vi "ForecastData Randomize Short.vi"(10 "DeviceID":T2) -> (3 "ForecastData_Short Array out":T1[](array[typedef]))   [LabVIEW 2018, in "IED Test Framework.lvlib" / "IED Test.lvclass"]
uses:
  IED Test.lvclass
  <vilib>/ORNL/CSEISMIC DDS/CSEISMIC DDS Base/Data Types/Controls/DeviceID.ctl
  <vilib>/ORNL/CSEISMIC DDS/CSEISMIC DDS Base/Data Types/ForecastData_Data.ctl
  <vilib>/ORNL/CSEISMIC DDS/CSEISMIC DDS Base/CSEISMIC DDS.lvclass
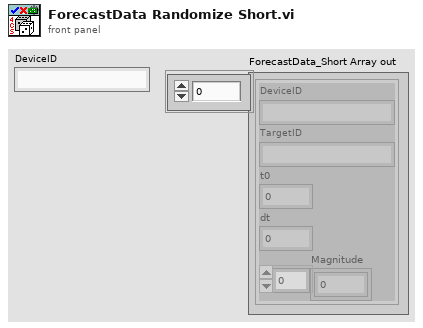
[diagram p1: front panel]
types:
  T1 = typedef "CSEISMIC DDS.lvlib/CSEISMIC DDS.lvclass/ForecastData_Data.ctl" = cluster{"DeviceID":T2, "TargetID":T2, "t0":dbl, "dt":dbl, "Magnitude":dbl[]}
  T2 = typedef "CSEISMIC DDS.lvlib/CSEISMIC DDS.lvclass/DeviceID.ctl" = string
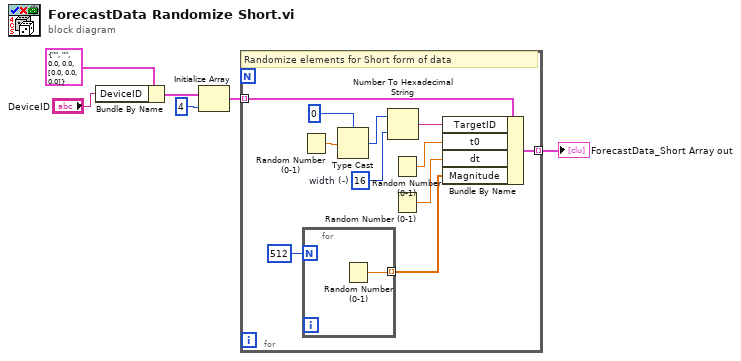
[diagram p0: block diagram]
diagram:
  n1 = Bundle By Name(cluster=T1 {"DeviceID"="", "TargetID"="", "t0"=0.0, "dt"=0.0, "Magnitude"=[0.0, 0.0, 0.0]} ("ForecastData"), "DeviceID"="DeviceID") -> (w6:T1)
  n2 = Initialize Array(w6, 4 ("dimension size")) -> (w3:T1[])
  n3 = for {
    tunnel: w3 -> [w17] mode=indexing
    tunnel: [w16] -> w1 mode=indexing
    w7 = i16 16  # width (-)
    # "Randomize elements for Short form of data"
    n4 = Random Number (0-1)() -> (number: 0 to 1=w11:dbl)
    n5 = for {
      N: 512 -> [_]
      tunnel: [w18] -> w12 mode=indexing
      n6 = Random Number (0-1)() -> (number: 0 to 1=w18:dbl)
    }
    n7 = Type Cast(type=u64 0 ("TargetID"), x=w11) -> (*(type *) &x=w9:u64)
    n8 = Number To Hexadecimal String(1:w7, 2:w9) -> (0:w8:string)
    n9 = Random Number (0-1)() -> (number: 0 to 1=w15:dbl)
    n10 = Random Number (0-1)() -> (number: 0 to 1=w14:dbl)
    n11 = Bundle By Name(cluster=w17, "TargetID"=w8, "t0"=w15, "dt"=w14, "Magnitude"=w12) -> (w16:T1)
  }
  "ForecastData_Short Array out" <- w1
